vi "ClientSrv Example Server.vi"   [LabVIEW 2012]
doc: "This is the top-level VI that starts a server application. It bootstraps LuaVIEW and hands over control to a series of initialisation scripts that define what the application does. The first script is named \"bootstrap.lua\" and is read from a \"resources\" directory located respectively in the same directory as this VI or inside the application directory, depending on whether this VI is run under the development system or as a built application.\n\nWhen building a server application, this is the main VI to include in the build. In addition you will need to include any dynamically loaded VIs, functions, modules, and plug-ins that are used by the server's scripts."
uses:
  subvis/private/glb_ClientSrv Globals.vi
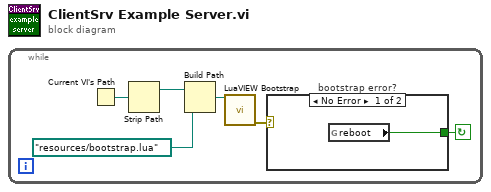
[diagram p0: block diagram]
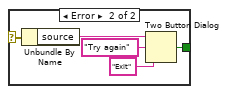
[diagram p2: hidden frame]
diagram:
  n1 = while {
    stop <- w2 continue-if-true
    n2 = Current VI's Path() -> (path=w1:path)
    n3 = Strip Path(path=w1) -> (stripped path=w4:path)  [unwired: 1 out]
    n4 = Build Path(base path=w4, name or relative path=path "resources/bootstrap.lua" ("script file or name (no name)")) -> (appended path=w5:path)
    n5 = call "LuaVIEW Bootstrap.vi"("script file or name (no name)"=w5) -> ("error out"=w3:errorcluster)  [unwired: 14 in]
    n6 = case "bootstrap error?" shown="No Error" w3 {
      selector: w3 -> [_ w12]
      tunnel: [w7 w8] -> w2
      frame No Error {
        n7 = global read "glb_ClientSrv Globals.vi" "reboot"() -> (w7:bool)
      }
      frame Error {
        n8 = Unbundle By Name(w12) -> ("source"=w11:string)
        n9 = Two Button Dialog(message=w11, 1:"Exit" ("F button name (\"Cancel\")"), 2:"Try again" ("T button name (\"OK\")")) -> (T button?=w8:bool)
      }
    }
  }
